vi "BRig_Host__Loop_Consumer_RunState__closedLoop_storeData_currentData.vi"(5 "input_dataExp":u16[](array[numeric]), 7 "input_dataLC":u16[](array[numeric]), 8 "input_updateID":u16, 9 "input_idx":i32[](array[numeric]), 10 "input_dataTS":u16[][](array[numeric]), 11 "input_dataPlot":u16[][](array[numeric])) -> (0 "output_filepath_dataTS":path, 1 "output_dataTS":bool, 2 "output_filepath_dataPlot":path, 3 "output_dataPlot":bool, 4 "output_filepath_dataExp":path, 6 "output_filepath_dataLC":path)   [LabVIEW 2014]
uses:
  <vilib>/Utility/file.llb/Write To Spreadsheet File (DBL).vi
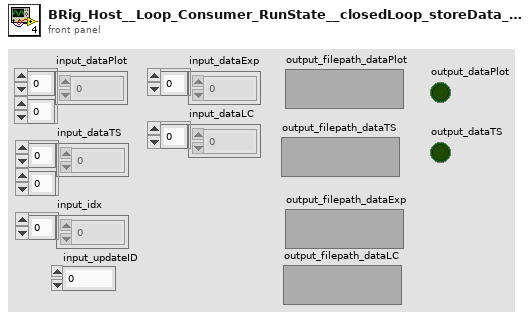
[diagram p1: front panel]
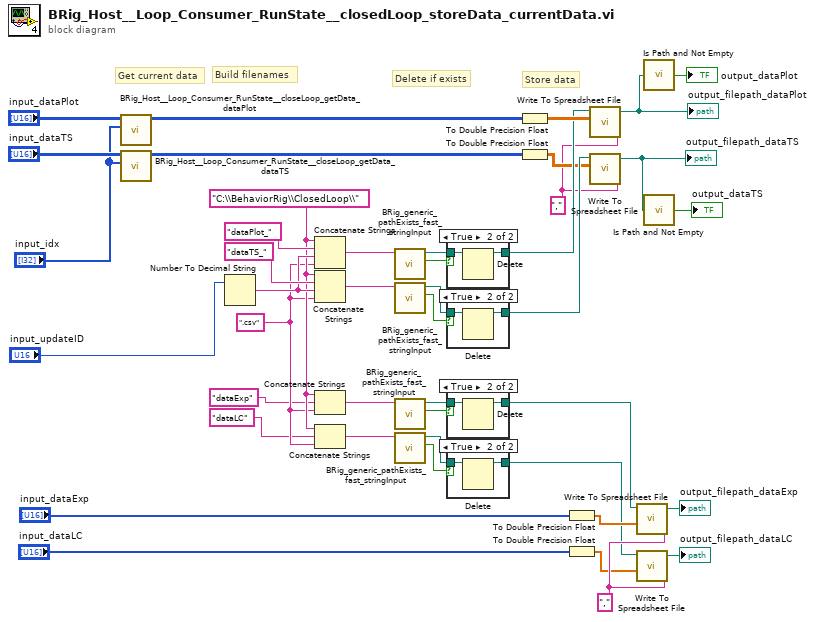
[diagram p0: block diagram]
diagram:
  w9 = "," ("delimiter (\\t)")
  w24 = "," ("delimiter (\\t)")
  w12 = ".csv"
  w13 = "C:\\BehaviorRig\\ClosedLoop\\"
  # "Delete if exists"
  # "Build filenames"
  # "Store data"
  # "Get current data"
  n1 = call "BRig_Host__Loop_Consumer_RunState__closeLoop_getData_dataPlot.vi"("input_idx"="input_idx", "input_dataPlot"="input_dataPlot") -> ("output_dataPlot"=w30:u16[][])  [unwired: 9 in]
  n2 = call "BRig_Host__Loop_Consumer_RunState__closeLoop_getData_dataTS.vi"("input_idx"="input_idx", "input_dataTS"="input_dataTS") -> ("output_dataTS"=w26:u16[][])  [unwired: 9 in]
  n3 = Number To Decimal String(number="input_updateID") -> (decimal integer string=w38:string)  [unwired: 1 in]
  n4 = Concatenate Strings(w13, "dataPlot_", w38, w12) -> (w37:string)
  n5 = Concatenate Strings(w13, "dataTS_", w38, w12) -> (w36:string)
  n6 = Concatenate Strings(w13, "dataExp", w12) -> (w19:string)
  n7 = Concatenate Strings(w13, "dataLC", w12) -> (w18:string)
  n8 = call "BRig_generic_pathExists_fast_stringInput.vi"("input_filePath"=w37) -> ("output_Iexist"=w35:bool, "output_filePath"=w34:path)  [unwired: 8 in, 1 out]
  n9 = call "BRig_generic_pathExists_fast_stringInput.vi"("input_filePath"=w36) -> ("output_Iexist"=w32:bool, "output_filePath"=w33:path)  [unwired: 8 in, 1 out]
  n10 = call "BRig_generic_pathExists_fast_stringInput.vi"("input_filePath"=w19) -> ("output_Iexist"=w17:bool, "output_filePath"=w16:path)  [unwired: 8 in, 1 out]
  n11 = call "BRig_generic_pathExists_fast_stringInput.vi"("input_filePath"=w18) -> ("output_Iexist"=w14:bool, "output_filePath"=w15:path)  [unwired: 8 in, 1 out]
  n12 = case shown="True" w35 {
    tunnel: w34 -> [w44 w46]
    tunnel: [w44 w45] -> w28
    frame False {
    }
    frame True {
      n13 = Delete(path (use dialog)=w46) -> (deleted path=w45:path)  [unwired: 4 in, 2 out]
    }
  }
  n14 = case shown="True" w32 {
    tunnel: w33 -> [w47 w49]
    tunnel: [w47 w48] -> w27
    frame False {
    }
    frame True {
      n15 = Delete(path (use dialog)=w49) -> (deleted path=w48:path)  [unwired: 4 in, 2 out]
    }
  }
  n16 = case shown="True" w17 {
    tunnel: w16 -> [w50 w52]
    tunnel: [w50 w51] -> w4
    frame False {
    }
    frame True {
      n17 = Delete(path (use dialog)=w52) -> (deleted path=w51:path)  [unwired: 4 in, 2 out]
    }
  }
  n18 = case shown="True" w14 {
    tunnel: w15 -> [w53 w55]
    tunnel: [w53 w54] -> w1
    frame False {
    }
    frame True {
      n19 = Delete(path (use dialog)=w55) -> (deleted path=w54:path)  [unwired: 4 in, 2 out]
    }
  }
  n20 = To Double Precision Float(number=w30) -> (double precision float=w29:dbl[][])
  n21 = To Double Precision Float(number=w26) -> (double precision float=w25:dbl[][])
  n22 = To Double Precision Float(number="input_dataExp") -> (double precision float=w6:dbl[])
  n23 = To Double Precision Float(number="input_dataLC") -> (double precision float=w5:dbl[])
  n24 = call-poly <vilib>:"Write To Spreadsheet File.vi"("delimiter (\\t)"=w24, "2D data"=w29, "file path (dialog if empty)"=w28) -> ("new file path (Not A Path if cancelled)"=w23:path)  [unwired: 5 in]
  "output_filepath_dataPlot" <- w23
  n25 = call-poly <vilib>:"Write To Spreadsheet File.vi"("delimiter (\\t)"=w24, "2D data"=w25, "file path (dialog if empty)"=w27) -> ("new file path (Not A Path if cancelled)"=w20:path)  [unwired: 5 in]
  "output_filepath_dataTS" <- w20
  n26 = call-poly <vilib>:"Write To Spreadsheet File.vi"("delimiter (\\t)"=w9, "1D data"=w6, "file path (dialog if empty)"=w4) -> ("new file path (Not A Path if cancelled)"=→"output_filepath_dataExp":path)  [unwired: 5 in]
  n27 = call-poly <vilib>:"Write To Spreadsheet File.vi"("delimiter (\\t)"=w9, "1D data"=w5, "file path (dialog if empty)"=w1) -> ("new file path (Not A Path if cancelled)"=→"output_filepath_dataLC":path)  [unwired: 5 in]
  n28 = call <vilib>:"Is Path and Not Empty.vi"("path"=w23) -> ("Is Path and Not Empty?"=→"output_dataPlot":bool)  [unwired: 4 in]
  n29 = call <vilib>:"Is Path and Not Empty.vi"("path"=w20) -> ("Is Path and Not Empty?"=→"output_dataTS":bool)  [unwired: 4 in]
